vi "Add Package to SystemLink Feed (By ID).vi"(0 "SystemLink repo in":T1, 5 "feed name in":string, 7 "package ID":string, 9 "timeout (ms) (10000)":u32=10000, 11 "error in (no error)":errorcluster) -> (4 "SystemLink repo out":T1, 6 "feed name out":string, 10 "timed out?":bool, 15 "error out":errorcluster)   [LabVIEW 2017, in "SystemLink_Repo_API.lvlib"]
doc: "Adds the package (that corresponds to the specified Package ID) to the specified feed, and waits for completion.\n\nError Handling:\nReturns an error if the specified feed or package ID does not exist in the SystemLink repository."
uses:
  systemlink repo.ctl
  <vilib>/httpClient/ClientHandle.ctl
  11e22a70-f141-46f2-99f4-c1a96e6a99a8.vi
  <vilib>/JDP Science/JSONtext/Find Item.vi
  <vilib>/JDP Science/JSONtext/String Subset.vi
  <vilib>/httpClient/POSTBuffer.vi
  <vilib>/JDP Science/JSONtext/Parsing/Parse Full Path or Item Name.vi
  <vilib>/JDP Science/JSONtext/Offset/Find Item Locations by Path.vi
  <vilib>/JDP Science/JSONtext/JSON text to Variant.vi
  SystemLink_Repo_API.lvlib
  <vilib>/httpClient/LabVIEWHTTPClient.lvlib
panel:
  out "job ID":string
  out "body":string
  out "headers":string
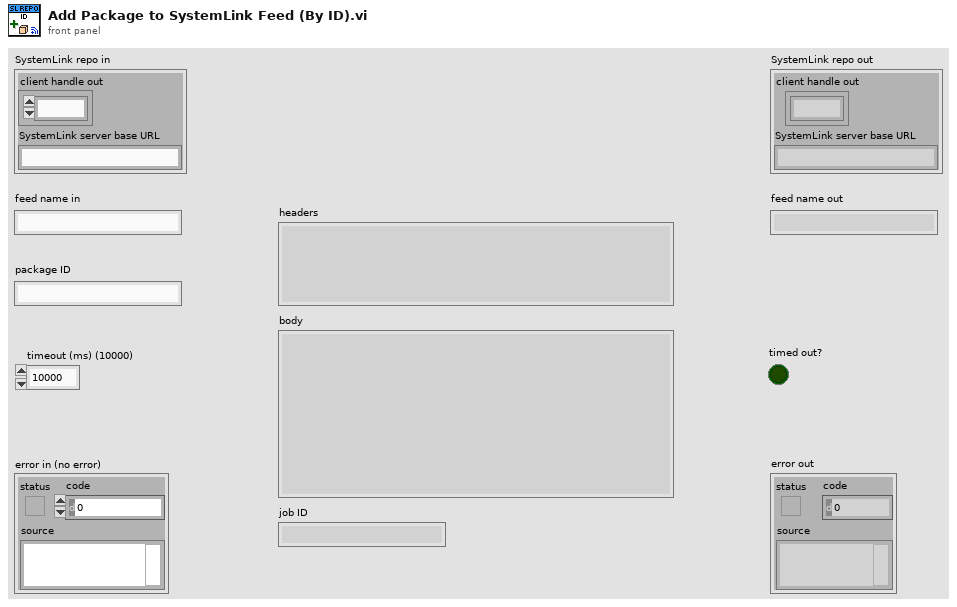
[diagram p1: front panel]
types:
  T1 = typedef "SystemLink_Repo_API.lvlib/systemlink repo.ctl" = cluster{"client handle out":T2, "SystemLink server base URL":string}
  T2 = typedef "LabVIEWHTTPClient.lvlib/ClientHandle.ctl" = refnum<k1>
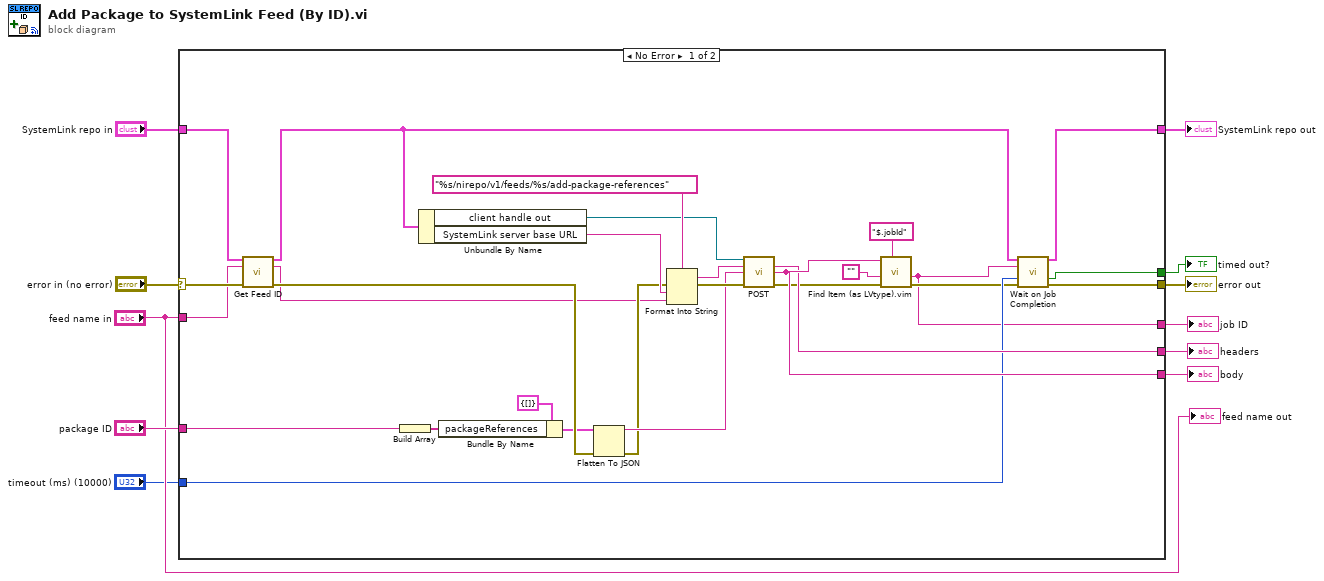
[diagram p0: block diagram]
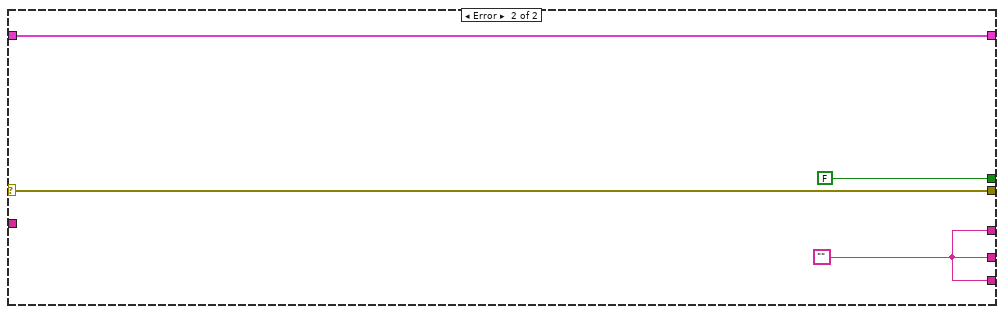
[diagram p2: hidden frame]
diagram:
  n1 = case shown="No Error" "error in (no error)" {
    selector: "error in (no error)" -> [w32 w43]
    tunnel: "SystemLink repo in" -> [w30 w42]
    tunnel: [w36 w43] -> w9
    tunnel: [w39 w40] -> w8
    tunnel: [w38 w40] -> w7
    tunnel: [w35 w42] -> w6
    tunnel: "feed name in" -> [w15 _]
    tunnel: "package ID" -> [w37 _]
    tunnel: "timeout (ms) (10000)" -> [w34 _]
    tunnel: [w33 FALSE ("timed out?")] -> w2
    tunnel: [w12 w40] -> w1
    frame No Error {
      n2 = call "Get Feed ID.vi"("SystemLink repo in"=w30, "feed name"=w15, "error in (no error)"=w32) -> ("SystemLink repo out"=w29:T1, "feed ID"=w16:string, "error out"=w31:errorcluster)  [unwired: 10 in]
      n3 = Build Array(w37) -> (w20:string[])
      n4 = Unbundle By Name(w29) -> ("client handle out"=w26:T2, "SystemLink server base URL"=w22:string)
      n5 = Bundle By Name(cluster=cluster{"packageReferences":string[]} {"packageReferences"=[]}, "packageReferences"=w20) -> (w19:cluster{"packageReferences":string[]})
      n6 = Flatten To JSON(anything=w19, error in (no error)=w31) -> (JSON string=w18:string, 11:w17:errorcluster)  [unwired: 1 in]
      n7 = Format Into String(format string="%s/nirepo/v1/feeds/%s/add-package-references", error in=w17, w22, w16) -> (resulting string=w27:string, error out=w25:errorcluster)  [unwired: 1 in]
      n8 = call-poly <vilib>:"POST.vi"("client handle"=w26, "url"=w27, "buffer"=w18, "error in (no error)"=w25) -> ("headers"=w38:string, "body"=w39:string, "error out"=w14:errorcluster)  [unwired: 8 in, 1 out]
      n9 = call "Find Item (as LVtype).vim"("$Path or Item Name"="$.jobId", "error in (no error)"=w14, "Data Type and Default Value"="", "JSON"=w39) -> ("error out"=w13:errorcluster, "Data"=w12:string)  [unwired: 4 in, 2 out]
      n10 = call "Wait on Job Completion.vi"("SystemLink repo in"=w29, "job ID"=w12, "timeout (ms) (10000)"=w34, "error in (no error)"=w13) -> ("SystemLink repo out"=w35:T1, "timed out?"=w33:bool, "error out"=w36:errorcluster)  [unwired: 8 in, 1 out]
    }
    frame Error {
      w40 = "" ("headers")
    }
  }
  "error out" <- w9
  "SystemLink repo out" <- w6
  "headers" <- w7
  "body" <- w8
  "timed out?" <- w2
  "job ID" <- w1
  "feed name out" <- "feed name in"
